vi "lamp-IsPort.vi"(8 "error in (no error)":errorcluster, 11 "Lamp":refnum<vi>) -> (0 "error out":errorcluster, 2 "Boolean":bool, 3 "Lamp":refnum<vi>)   [LabVIEW 2016]
uses:
  controls/lamp.ctl
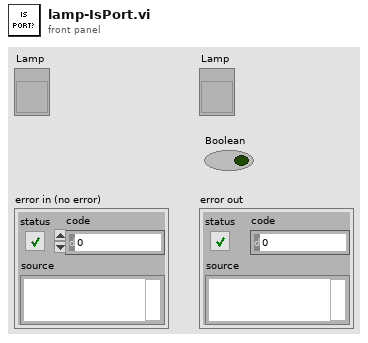
[diagram p1: front panel]
types:
  T1 = typedef "lamp.ctl" = cluster{"Port":refnum<visa-resource-name>, "Power":u16, "Is Conected?":bool, "ON":bool, "Open":bool, "Save":bool, "Model":string}
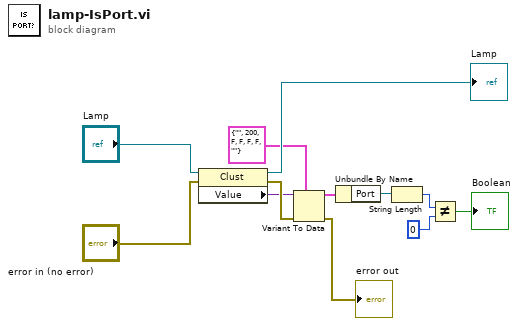
[diagram p0: block diagram]
diagram:
  n1 = property class="Clust"(reference="Lamp", error in="error in (no error)") -> (reference out=→"Lamp":refnum<vi>, error out=w4:errorcluster, "Value"=w3:variant)
  n2 = Variant To Data(error in=w4, type=T1 {"Port"="", "Power"=200, "Is Conected?"=FALSE, "ON"=FALSE, "Open"=FALSE, "Save"=FALSE, "Model"=""} ("Lamp"), Variant=w3) -> (data=w6:T1, error out=→"error out":errorcluster)
  n3 = Unbundle By Name(w6) -> ("Port"=w7:refnum<visa-resource-name>)
  n4 = String Length(string=w7) -> (length=w8:i32)
  n5 = Not Equal?(x=w8, y=0) -> (x != y?=→"Boolean":bool)
